vi "Count True Booleans.vi"(4 "Boolean Array":bool[](array[boolean])) -> (1 "Number of True":i32)   [LabVIEW 2011]
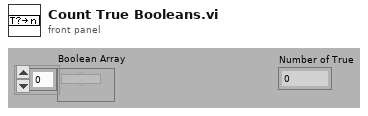
[diagram p1: front panel]
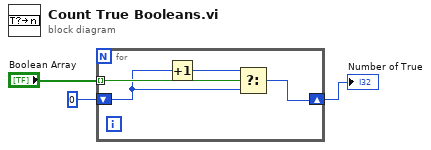
[diagram p0: block diagram]
diagram:
  n1 = for {
    tunnel: "Boolean Array" -> [w7] mode=indexing
    shift-right: [w4] -> w1
    shift-left: 0 -> [w6]
    n2 = Increment(x=w6) -> (x+1=w5:i32)
    n3 = Select(t=w5, s=w7, f=w6) -> (s? t:f=w4:i32)
  }
  "Number of True" <- w1
